vi "VSG25A_StepSweep.vi"(3 "Error In":errorcluster, 4 "Sweep Params In":T1={"Start Freq"=0.6, "Stop Freq"=1.0, "Start Hz"=3, "Stop Hz"=3, "Step Freq"=100.0, "Step Hz"=2, "Amplitude"=-10.0, "Dwell Time"=1000.0} {"Start Hz" items=["Hz", "kHz", "MHz", "GHz"]; "Stop Hz" items=["Hz", "kHz", "MHz", "GHz"]; "Step Hz" items=["Hz", "kHz", "MHz", "GHz"]}, 5 "Device Handle In":i32) -> (0 "Error Out":errorcluster, 2 "Device Handle Out":i32)   [LabVIEW 2014]
uses:
  Frequency Hertz.ctl
  Sweep Cluster.ctl
  sg_lib/VSG25A.lvlib
panel:
  out "Sweep Params Out":T1={"Start Freq"=1.0, "Stop Freq"=2.0, "Start Hz"=3, "Stop Hz"=3, "Step Freq"=100.0, "Step Hz"=2, "Amplitude"=-10.0, "Dwell Time"=100.0} {"Start Hz" items=["Hz", "kHz", "MHz", "GHz"]; "Stop Hz" items=["Hz", "kHz", "MHz", "GHz"]; "Step Hz" items=["Hz", "kHz", "MHz", "GHz"]}
  in  "RF On":bool
  in  "Step Freq Hz":T2 items=["Hz", "kHz", "MHz", "GHz"]
  in  "Stop Freq Hz":T2 items=["Hz", "kHz", "MHz", "GHz"]
  in  "Start Freq Hz":T2 items=["Hz", "kHz", "MHz", "GHz"]
  in  "Amplitude (dBm)":dbl
  out "Sweep Time":dbl
  out "Frequency Span":dbl
  in  "Dwell Time (mS)":dbl
  in  "Step Frequency":dbl
  in  "Stop Frequency":dbl
  in  "Start Frequency":dbl
  # "Step Sweep"
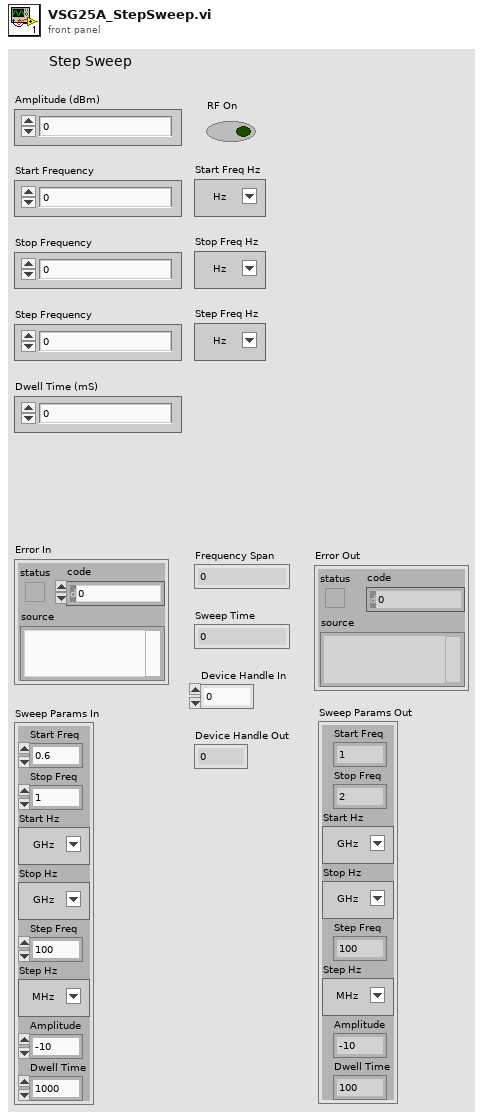
[diagram p1: front panel]
types:
  T1 = typedef "Sweep Cluster.ctl" = cluster{"Start Freq":dbl, "Stop Freq":dbl, "Start Hz":T2, "Stop Hz":T2, "Step Freq":dbl, "Step Hz":T2, "Amplitude":dbl, "Dwell Time":dbl}
  T2 = typedef "Frequency Hertz.ctl" = u16
  T3 = enum32{"Bad", "Idle", "Run top level", "Running"}
  T4 = enum16{"Check Amplitude", "Check Start Freq", "Check Stop Freq", "Check Step Freq", "Check Dwell Time", "Calc Freq Span", "Calc Sweep Time", "Stop RF", "Set Freq And Amp", "Set Sweep", "Finish", ""}
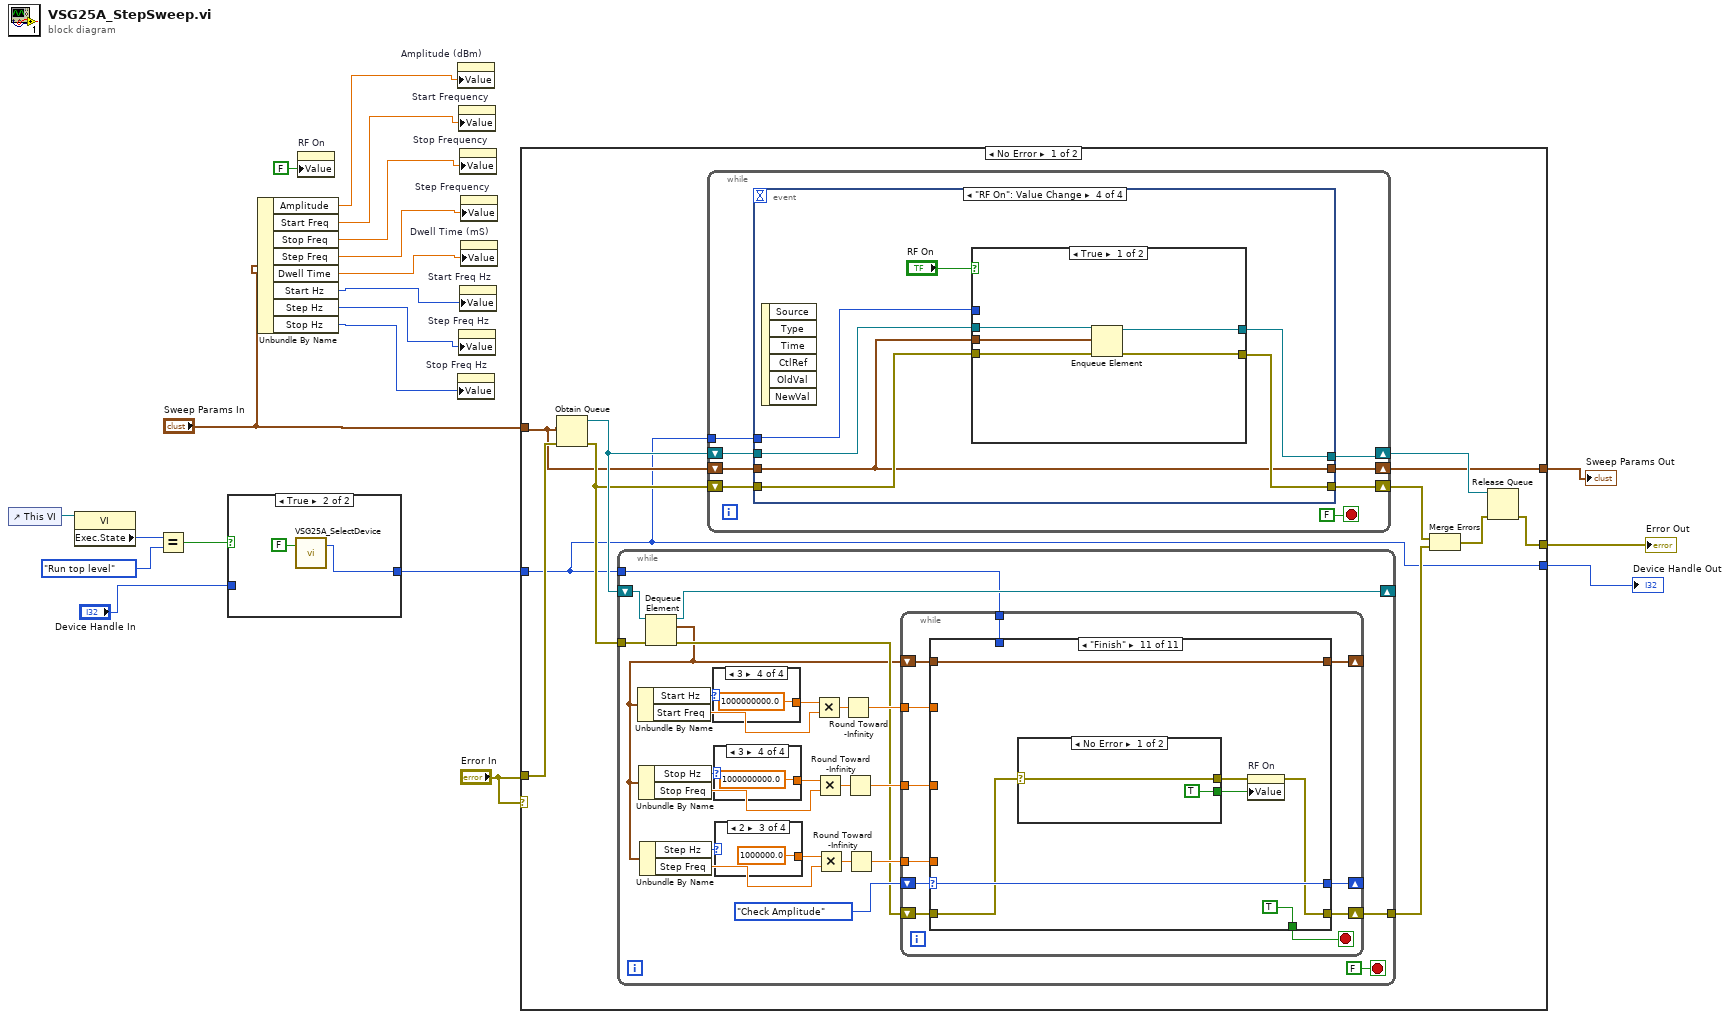
[diagram p0: block diagram]
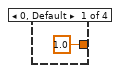
[diagram p3: hidden frame]
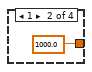
[diagram p4: hidden frame]
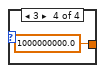
[diagram p5: hidden frame]
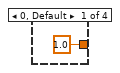
[diagram p6: hidden frame]
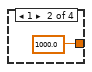
[diagram p7: hidden frame]
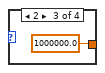
[diagram p8: hidden frame]
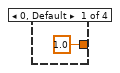
[diagram p9: hidden frame]
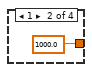
[diagram p10: hidden frame]
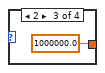
[diagram p11: hidden frame]
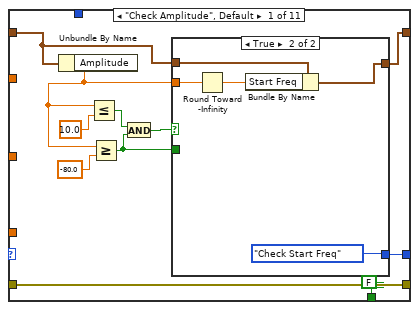
[diagram p12: hidden frame]
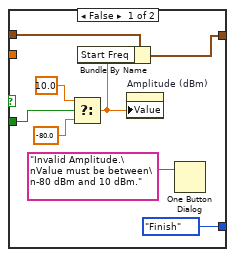
[diagram p13: hidden frame]
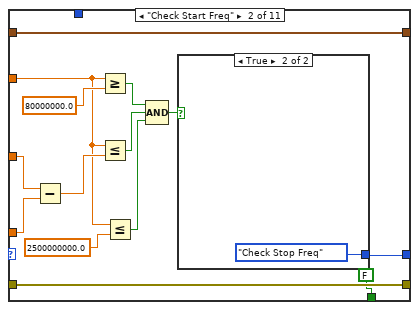
[diagram p14: hidden frame]
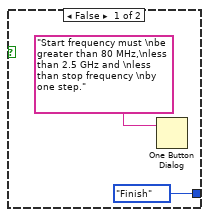
[diagram p15: hidden frame]
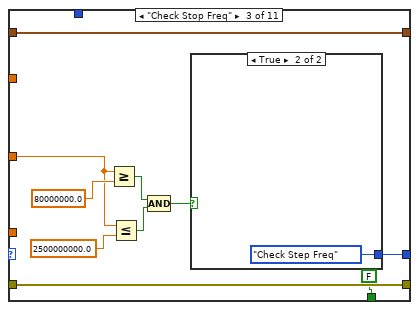
[diagram p16: hidden frame]
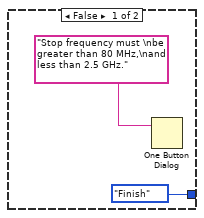
[diagram p17: hidden frame]
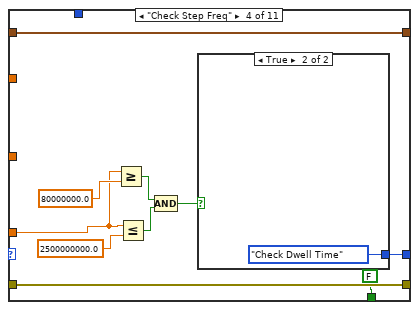
[diagram p18: hidden frame]
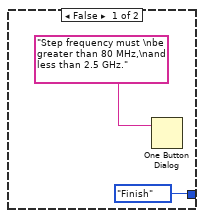
[diagram p19: hidden frame]
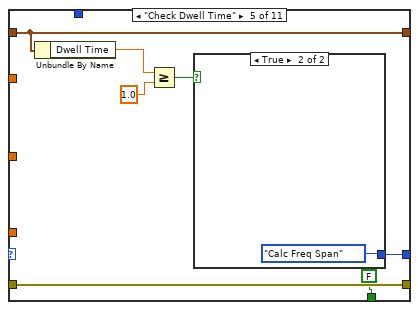
[diagram p20: hidden frame]
diagram:
  n1 = control-ref of="This VI"() -> (w6:refnum<vi>)
  n2 = property class="VI"(reference=w6) -> ("Exec.State"=w5:T3)  [unwired: 1 in, 2 out]
  n3 = Equal?(x=w5, y=T3."Run top level" ("Execution:State 2")) -> (x = y?=w3:bool)
  n4 = case shown="True" w3 {
    tunnel: [w21 w23] -> w2
    tunnel: "Device Handle In" -> [w21 _]
    frame False {
    }
    frame True {
      n5 = call "VSG25A_SelectDevice.vi"("AutoSel"=FALSE) -> ("deviceHandle"=w23:i32)  [unwired: 1 in, 1 out]
    }
  }
  n6 = Unbundle By Name("Sweep Params In") -> ("Amplitude"=w9:dbl, "Start Freq"=w10:dbl, "Stop Freq"=w11:dbl, "Step Freq"=w12:dbl, "Dwell Time"=w13:dbl, "Start Hz"=w14:T2, "Step Hz"=w15:T2, "Stop Hz"=w16:T2)
  n7 = property on="RF On" class="Bool (strict)"("Value"=FALSE ("RF On")) -> ()  [unwired: 2 in, 2 out]
  n8 = property on="Amplitude (dBm)" class="DigNum (strict)"("Value"=w9) -> ()  [unwired: 2 in, 2 out]
  n9 = property on="Stop Freq Hz" class="Ring (strict)"("Value"=w16) -> ()  [unwired: 2 in, 2 out]
  n10 = property on="Start Frequency" class="DigNum (strict)"("Value"=w10) -> ()  [unwired: 2 in, 2 out]
  n11 = property on="Step Freq Hz" class="Ring (strict)"("Value"=w15) -> ()  [unwired: 2 in, 2 out]
  n12 = property on="Stop Frequency" class="DigNum (strict)"("Value"=w11) -> ()  [unwired: 2 in, 2 out]
  n13 = property on="Start Freq Hz" class="Ring (strict)"("Value"=w14) -> ()  [unwired: 2 in, 2 out]
  n14 = property on="Step Frequency" class="DigNum (strict)"("Value"=w12) -> ()  [unwired: 2 in, 2 out]
  n15 = property on="Dwell Time (mS)" class="DigNum (strict)"("Value"=w13) -> ()  [unwired: 2 in, 2 out]
  n16 = case shown="No Error" "Error In" {
    tunnel: "Error In" -> [w27 w285]
    tunnel: [w30 w285] -> w19
    tunnel: "Sweep Params In" -> [w26 w283]
    tunnel: w2 -> [w25 w284]
    tunnel: [w25 w284] -> w18
    tunnel: [w24 w283] -> w7
    frame No Error {
      n17 = Obtain Queue(element data type=w26, error in (no error)=w27) -> (queue out=w29:refnum<queue>, error out=w28:errorcluster)  [unwired: 3 in, 1 out]
      n18 = while {
        tunnel: w28 -> [w58]
        shift-right: [w56] -> _
        shift-left: w29 -> [w57]
        tunnel: w25 -> [w37]
        tunnel: [w36] -> w33
        stop <- FALSE stop-if-true
        n19 = Dequeue Element(queue=w57, error in (no error)=w58) -> (queue out=w56:refnum<queue>, element=w38:T1, error out=w39:errorcluster)  [unwired: 1 in, 1 out]
        n20 = Unbundle By Name(w38) -> ("Start Hz"=w52:T2, "Start Freq"=w53:dbl)
        n21 = Unbundle By Name(w38) -> ("Stop Hz"=w51:T2, "Stop Freq"=w50:dbl)
        n22 = Unbundle By Name(w38) -> ("Step Hz"=w43:T2, "Step Freq"=w44:dbl)
        n23 = case shown="3" w52 {
          tunnel: [1.0 ("y") 1000.0 ("y") 1000000.0 ("y") 1000000000.0 ("y")] -> w54
          frame 0, Default {
          }
          frame 1 {
          }
          frame 2 {
          }
          frame 3 {
          }
        }
        n24 = case shown="3" w51 {
          tunnel: [1.0 ("y") 1000.0 ("y") 1000000.0 ("y") 1000000000.0 ("y")] -> w49
          frame 0, Default {
          }
          frame 1 {
          }
          frame 2 {
          }
          frame 3 {
          }
        }
        n25 = case shown="2" w43 {
          tunnel: [1.0 ("y") 1000.0 ("y") 1000000.0 ("y") 1000000000.0 ("y")] -> w45
          frame 0, Default {
          }
          frame 1 {
          }
          frame 2 {
          }
          frame 3 {
          }
        }
        n26 = Multiply(x=w54, y=w53) -> (x*y=w48:dbl)
        n27 = Multiply(x=w49, y=w50) -> (x*y=w47:dbl)
        n28 = Multiply(x=w45, y=w44) -> (x*y=w46:dbl)
        n29 = Round Toward -Infinity(1:w48) -> (0:w42:dbl)
        n30 = Round Toward -Infinity(1:w47) -> (0:w41:dbl)
        n31 = Round Toward -Infinity(1:w46) -> (0:w40:dbl)
        n32 = while {
          shift-right: [w79] -> _
          shift-left: w38 -> [w80]
          shift-right: [w78] -> _
          shift-left: T4."Check Amplitude" -> [w81]
          tunnel: w42 -> [w77]
          tunnel: w41 -> [w76]
          tunnel: w40 -> [w75]
          tunnel: w37 -> [w73]
          shift-right: [w72] -> w36
          shift-left: w39 -> [w74]
          stop <- w71 stop-if-true
          n33 = case shown="\"Finish\"" w81 {
            selector: w81 -> [_ _ _ _ _ _ _ _ _ _ w202]
            tunnel: w80 -> [w86 w107 w125 w138 w151 w161 w171 w175 w182 w190 w197]
            tunnel: [w85 w107 w125 w138 w151 w161 w171 w175 w182 w190 w197] -> w79
            tunnel: [w84 w115 w126 w139 w152 T4."Calc Sweep Time" T4."Stop RF" T4."Set Freq And Amp" T4."Set Sweep" T4."Finish" w202] -> w78
            tunnel: w77 -> [_ w113 _ _ _ w164 _ _ _ _ _]
            tunnel: w76 -> [_ w118 w130 _ _ w165 _ _ _ _ _]
            tunnel: w75 -> [_ w117 _ w140 _ _ _ _ _ _ _]
            tunnel: w74 -> [w83 w108 w124 w137 w150 w160 w170 w178 w187 w194 w201]
            tunnel: w73 -> [_ _ _ _ _ _ _ w176 w184 w195 _]
            tunnel: [w83 w108 w124 w137 w150 w160 w170 w177 w186 w193 w199] -> w72
            tunnel: [FALSE FALSE FALSE FALSE FALSE FALSE FALSE FALSE FALSE FALSE TRUE] -> w71
            frame "Check Amplitude", Default {
              n34 = Unbundle By Name(w86) -> ("Amplitude"=w87:dbl)
              n35 = Less Or Equal?(x=w87, y=10.0) -> (x <= y?=w91:bool)
              n36 = Greater Or Equal?(x=w87, y=-80.0) -> (x >= y?=w88:bool)
              n37 = And(x=w91, y=w88) -> (x .and. y?=w92:bool)
              n38 = case shown="True" w92 {
                tunnel: w88 -> [w100 _]
                tunnel: w87 -> [_ w104]
                tunnel: w86 -> [w97 w103]
                tunnel: [w96 w102] -> w85
                tunnel: [T4."Finish" T4."Check Start Freq"] -> w84
                frame False {
                  n39 = Select(t=10.0, s=w100, f=-80.0) -> (s? t:f=w95:dbl)
                  n40 = Bundle By Name(cluster=w97, "Start Freq"=w95) -> (w96:T1)
                  n41 = property on="Amplitude (dBm)" class="DigNum (strict)"("Value"=w95) -> ()  [unwired: 2 in, 2 out]
                  n42 = One Button Dialog(message="Invalid Amplitude.\nValue must be between\n-80 dBm and 10 dBm.") -> ()  [unwired: 1 in, 1 out]
                }
                frame True {
                  n43 = Round Toward -Infinity(1:w104) -> (0:w105:dbl)
                  n44 = Bundle By Name(cluster=w103, "Start Freq"=w105) -> (w102:T1)
                }
              }
            }
            frame "Check Start Freq" {
              n45 = Subtract(x=w118, y=w117) -> (x-y=w116:dbl)
              n46 = Greater Or Equal?(x=w113, y=80000000.0) -> (x >= y?=w111:bool)
              n47 = Less Or Equal?(x=w113, y=w116) -> (x <= y?=w110:bool)
              n48 = Less Or Equal?(x=w113, y=2500000000.0) -> (x <= y?=w109:bool)
              n49 = Compound Arithmetic op=AND(w111, w110, w109) -> (w112:bool)
              n50 = case shown="True" w112 {
                tunnel: [T4."Finish" T4."Check Stop Freq"] -> w115
                frame False {
                  n51 = One Button Dialog(message="Start frequency must \nbe greater than 80 MHz,\nless than 2.5 GHz and \nless than stop frequency \nby one step.") -> ()  [unwired: 1 in, 1 out]
                }
                frame True {
                }
              }
            }
            frame "Check Stop Freq" {
              n52 = Greater Or Equal?(x=w130, y=80000000.0) -> (x >= y?=w129:bool)
              n53 = Less Or Equal?(x=w130, y=2500000000.0) -> (x <= y?=w128:bool)
              n54 = Compound Arithmetic op=AND(w129, w128) -> (w127:bool)
              n55 = case shown="True" w127 {
                tunnel: [T4."Finish" T4."Check Step Freq"] -> w126
                frame False {
                  n56 = One Button Dialog(message="Stop frequency must \nbe greater than 80 MHz,\nand less than 2.5 GHz.") -> ()  [unwired: 1 in, 1 out]
                }
                frame True {
                }
              }
            }
            frame "Check Step Freq" {
              n57 = Greater Or Equal?(x=w140, y=80000000.0) -> (x >= y?=w143:bool)
              n58 = Less Or Equal?(x=w140, y=2500000000.0) -> (x <= y?=w142:bool)
              n59 = Compound Arithmetic op=AND(w143, w142) -> (w141:bool)
              n60 = case shown="True" w141 {
                tunnel: [T4."Finish" T4."Check Dwell Time"] -> w139
                frame False {
                  n61 = One Button Dialog(message="Step frequency must \nbe greater than 80 MHz,\nand less than 2.5 GHz.") -> ()  [unwired: 1 in, 1 out]
                }
                frame True {
                }
              }
            }
            frame "Check Dwell Time" {
              n62 = Unbundle By Name(w151) -> ("Dwell Time"=w155:dbl)
              n63 = Greater Or Equal?(x=w155, y=1.0) -> (x >= y?=w153:bool)
              n64 = case shown="True" w153 {
                tunnel: [T4."Finish" T4."Calc Freq Span"] -> w152
                frame False {
                  n65 = One Button Dialog(message="Dwell time must be greater \nthan 1 milliSecond.") -> ()  [unwired: 1 in, 1 out]
                }
                frame True {
                }
              }
            }
            frame "Calc Freq Span" {
              n66 = Subtract(x=w165, y=w164) -> (x-y=→"Frequency Span":dbl)
            }
            frame "Calc Sweep Time" {
              n67 = Unbundle By Name(w171) -> ("Dwell Time"=w168:dbl)
              n68 = Divide(x=w168, y=1000.0) -> (x/y=w166:dbl)
              n69 = Round Toward -Infinity(1:w166) -> (0:→"Sweep Time":dbl)
            }
            frame "Stop RF" {
              n70 = call "sg RF Off.vi"("error in (no error)"=w178, "device"=w176) -> ("error out"=w177:errorcluster)  [unwired: 8 in, 1 out]
            }
            frame "Set Freq And Amp" {
              n71 = Unbundle By Name(w182) -> ("Amplitude"=w185:dbl)
              n72 = call "sg Set Frequency Amplitude.vi"("error in (no error)"=w187, "amplitude"=w185, "frequency"=800000000.0, "device"=w184) -> ("error out"=w186:errorcluster)  [unwired: 6 in, 1 out]
            }
            frame "Set Sweep" {
              n73 = property on="Sweep Time" class="DigNum (strict)" props=["Value"]() -> ()  [unwired: 2 in, 3 out]
              n74 = property on="Frequency Span" class="DigNum (strict)"() -> ("Value"=w192:dbl)  [unwired: 2 in, 2 out]
              n75 = call "sg Set Sweep.vi"("error in (no error)"=w194, "span"=5.0, "time"=w192, "device"=w195) -> ("error out"=w193:errorcluster)  [unwired: 6 in, 1 out]
            }
            frame "Finish" {
              n76 = case shown="No Error" w201 {
                selector: w201 -> [w204 w205]
                tunnel: [w204 w207] -> w200
                tunnel: [TRUE FALSE] -> w198
                frame No Error {
                }
                frame Error {
                  n77 = call <vilib>:"Simple Error Handler.vi"("error in (no error)"=w205) -> ("error out"=w206:errorcluster)  [unwired: 4 in, 4 out]
                  n78 = call <vilib>:"Clear Errors.vi"("error in (no error)"=w206) -> ("error out"=w207:errorcluster)  [unwired: 5 in, 1 out]
                }
              }
              n79 = property on="RF On" class="Bool (strict)"(error in=w200, "Value"=w198) -> (error out=w199:errorcluster)  [unwired: 1 in, 1 out]
            }
          }
        }
      }
      n80 = while {
        shift-right: [w214] -> w24
        shift-left: w26 -> [w215]
        shift-right: [w213] -> w34
        shift-left: w28 -> [w216]
        shift-right: [w211] -> w32
        shift-left: w29 -> [w212]
        tunnel: w25 -> [w209]
        stop <- FALSE stop-if-true
        n81 = event shown="[3] \"RF On\": Value Change" {
          selector: _ -> [_ _ _ _]
          dyn-events: _ -> [_ _ _ _]
          timeout: _ -> [_ _ _ _]
          tunnel: w216 -> [w217 w223 w255 w268]
          tunnel: w215 -> [w218 w232 w253 w267]
          tunnel: [w218 w233 w253 w267] -> w214
          tunnel: [w217 w222 w258 w271] -> w213
          tunnel: w212 -> [w219 w221 w252 w269]
          tunnel: [w219 w220 w252 w266] -> w211
          tunnel: w209 -> [_ _ w254 w265]
          event Timeout {
            n82 = event-data() -> ()  [unwired: 1 in, 3 out]
          }
          event "Amplitude (dBm)", "Dwell Time (mS)", "Start Frequency", "Stop Frequency", "Step Frequency": Value Change {
            n83 = event-data() -> ()  [unwired: 1 in, 6 out]
            n84 = property on="Start Freq Hz" class="Ring (strict)"() -> ("Value"=w226:T2)  [unwired: 2 in, 2 out]
            n85 = property on="Stop Freq Hz" class="Ring (strict)"() -> ("Value"=w224:T2)  [unwired: 2 in, 2 out]
            n86 = property on="Step Freq Hz" class="Ring (strict)"() -> ("Value"=w225:T2)  [unwired: 2 in, 2 out]
            n87 = property on="RF On" class="Bool (strict)"() -> ("Value"=w234:bool)  [unwired: 2 in, 2 out]
            n88 = case shown="False" w234 {
              tunnel: [w236 w242] -> w233
              tunnel: w232 -> [w236 w251]
              tunnel: "Amplitude (dBm)" -> [_ w250]
              tunnel: "Start Frequency" -> [_ w249]
              tunnel: "Stop Frequency" -> [_ w248]
              tunnel: "Step Frequency" -> [_ w247]
              tunnel: "Dwell Time (mS)" -> [_ w246]
              tunnel: w226 -> [_ w245]
              tunnel: w225 -> [_ w244]
              tunnel: w224 -> [_ w243]
              tunnel: w223 -> [w235 w241]
              tunnel: [w235 w240] -> w222
              tunnel: w221 -> [w237 w239]
              tunnel: [w237 w238] -> w220
              frame False {
              }
              frame True {
                n89 = Bundle By Name(cluster=w251, "Amplitude"=w250, "Start Freq"=w249, "Stop Freq"=w248, "Step Freq"=w247, "Dwell Time"=w246, "Start Hz"=w245, "Stop Hz"=w244, "Step Hz"=w243) -> (w242:T1)
                n90 = Enqueue Element(queue=w239, element=w242, error in (no error)=w241) -> (queue out=w238:refnum<queue>, error out=w240:errorcluster)  [unwired: 1 in, 1 out]
              }
            }
          }
          event Value Change {
            n91 = event-data() -> ()  [unwired: 1 in, 6 out]
            n92 = property on="RF On" class="Bool (strict)"(error in=w255) -> (error out=w256:errorcluster, "Value"=w257:bool)  [unwired: 1 in, 1 out]
            n93 = case shown="False" w257 {
              tunnel: [w259 w262] -> w258
              tunnel: w256 -> [w259 w261]
              tunnel: w254 -> [_ w260]
              frame False {
              }
              frame True {
                n94 = call "sg RF Off.vi"("error in (no error)"=w261, "device"=w260) -> ("error out"=w263:errorcluster)  [unwired: 8 in, 1 out]
                n95 = property on="RF On" class="Bool (strict)"(error in=w263, "Value"=FALSE ("RF On")) -> (error out=w262:errorcluster)  [unwired: 1 in, 1 out]
              }
            }
          }
          event "RF On": Value Change {
            n96 = event-data() -> ()  [unwired: 1 in, 6 out]
            n97 = case shown="True" "RF On" {
              tunnel: [w272 w280] -> w271
              tunnel: w269 -> [w276 w277]
              tunnel: w267 -> [w275 _]
              tunnel: w268 -> [w274 w279]
              tunnel: [w273 w277] -> w266
              tunnel: w265 -> [_ w278]
              frame True {
                n98 = Enqueue Element(queue=w276, element=w275, error in (no error)=w274) -> (queue out=w273:refnum<queue>, error out=w272:errorcluster)  [unwired: 1 in, 1 out]
              }
              frame False {
                n99 = call "sg RF Off.vi"("error in (no error)"=w279, "device"=w278) -> ("error out"=w281:errorcluster)  [unwired: 8 in, 1 out]
                n100 = property on="RF On" class="Bool (strict)"(error in=w281, "Value"=FALSE ("RF On")) -> (error out=w280:errorcluster)  [unwired: 1 in, 1 out]
              }
            }
          }
        }
      }
      n101 = Merge Errors(w34, w33) -> (w31:errorcluster)
      n102 = Release Queue(queue=w32, error in (no error)=w31) -> (error out=w30:errorcluster)  [unwired: 1 in, 2 out]
    }
    frame Error {
    }
  }
  "Error Out" <- w19
  "Device Handle Out" <- w18
  "Sweep Params Out" <- w7
